vi "Draw Conn Terminal.vi"(8 "Direction":T1, 9 "Rect":T2, 10 "Type Color":u32(colorbox), 11 "Picture  In":picture) -> (3 "Picture":picture)   [LabVIEW 2020, in "FlexBlock.xnode"]
uses:
  FlexBlock.xnode
  FlexBlocks/Terminal Direction.ctl
  FlexBlocks/FlexBlocks.lvlib
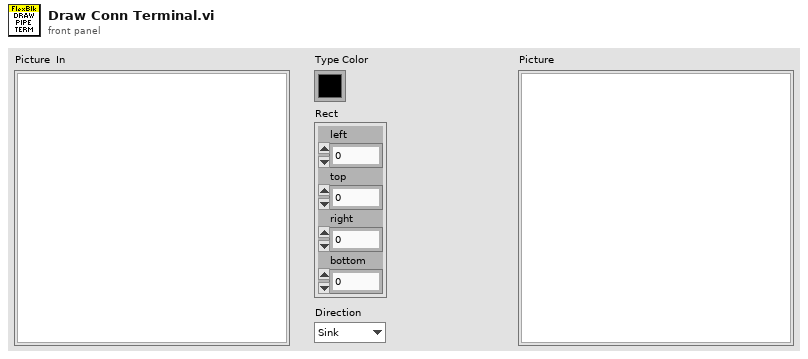
[diagram p1: front panel]
types:
  T1 = typedef "FlexBlocks.lvlib/Terminal Direction.ctl" = enum16{"Sink", "Source"}
  T2 = cluster{"left":i16, "top":i16, "right":i16, "bottom":i16}
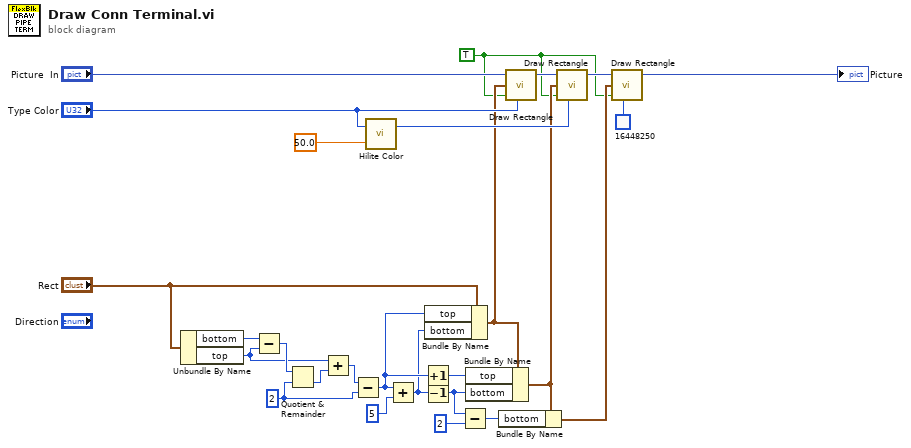
[diagram p0: block diagram]
diagram:
  w4 = TRUE ("fill?(F)")
  w16 = i16 2 ("y")
  n1 = Unbundle By Name("Rect") -> ("bottom"=w25:i16, "top"=w3:i16)
  n2 = Subtract(x=w25, y=w3) -> (x-y=w24:i16)
  n3 = Quotient & Remainder(x=w24, y=w16) -> (floor(x/y)=w2:i16)  [unwired: 1 out]
  n4 = Add(x=w3, y=w2) -> (x+y=w1:i16)
  n5 = Subtract(x=w1, y=w16) -> (x-y=w13:i16)
  n6 = call <vilib>:"Hilite Color.vi"("Percentage(30)"=50.0, "Color In"="Type Color") -> ("Hilite"=w18:u32)  [unwired: 1 out]
  n7 = Add(x=w13, y=i16 5) -> (x+y=w12:i16)
  n8 = Increment(x=w13) -> (x+1=w11:i16)
  n9 = Decrement(x=w12) -> (x-1=w9:i16)
  n10 = Bundle By Name(cluster="Rect", "top"=w13, "bottom"=w12) -> (w10:T2)
  n11 = Subtract(x=w9, y=i16 2) -> (x-y=w7:i16)
  n12 = Bundle By Name(cluster=w10, "top"=w11, "bottom"=w9) -> (w6:T2)
  n13 = Bundle By Name(cluster=w6, "bottom"=w7) -> (w5:T2)
  n14 = call <vilib>:"Draw Rectangle.vi"("picture"="Picture  In", "rect"=w10, "fill?(F)"=w4, "color(black)"="Type Color") -> ("new picture"=w21:picture)  [unwired: 5 in]
  n15 = call <vilib>:"Draw Rectangle.vi"("picture"=w21, "rect"=w6, "fill?(F)"=w4, "color(black)"=w18) -> ("new picture"=w20:picture)  [unwired: 5 in]
  n16 = call <vilib>:"Draw Rectangle.vi"("picture"=w20, "rect"=w5, "fill?(F)"=w4, "color(black)"=u32 16448250) -> ("new picture"=→"Picture":picture)  [unwired: 5 in]
